vi "PID Calibrator main.vi"() -> ()   [LabVIEW 2021]
panel:
  out "error out":errorcluster
  out "Waveform Chart":T1(graph)
  out "Numeric":i32
  out "remote port":u16
  out "remote address":string
  in  "stop":bool
  in  "port":u16
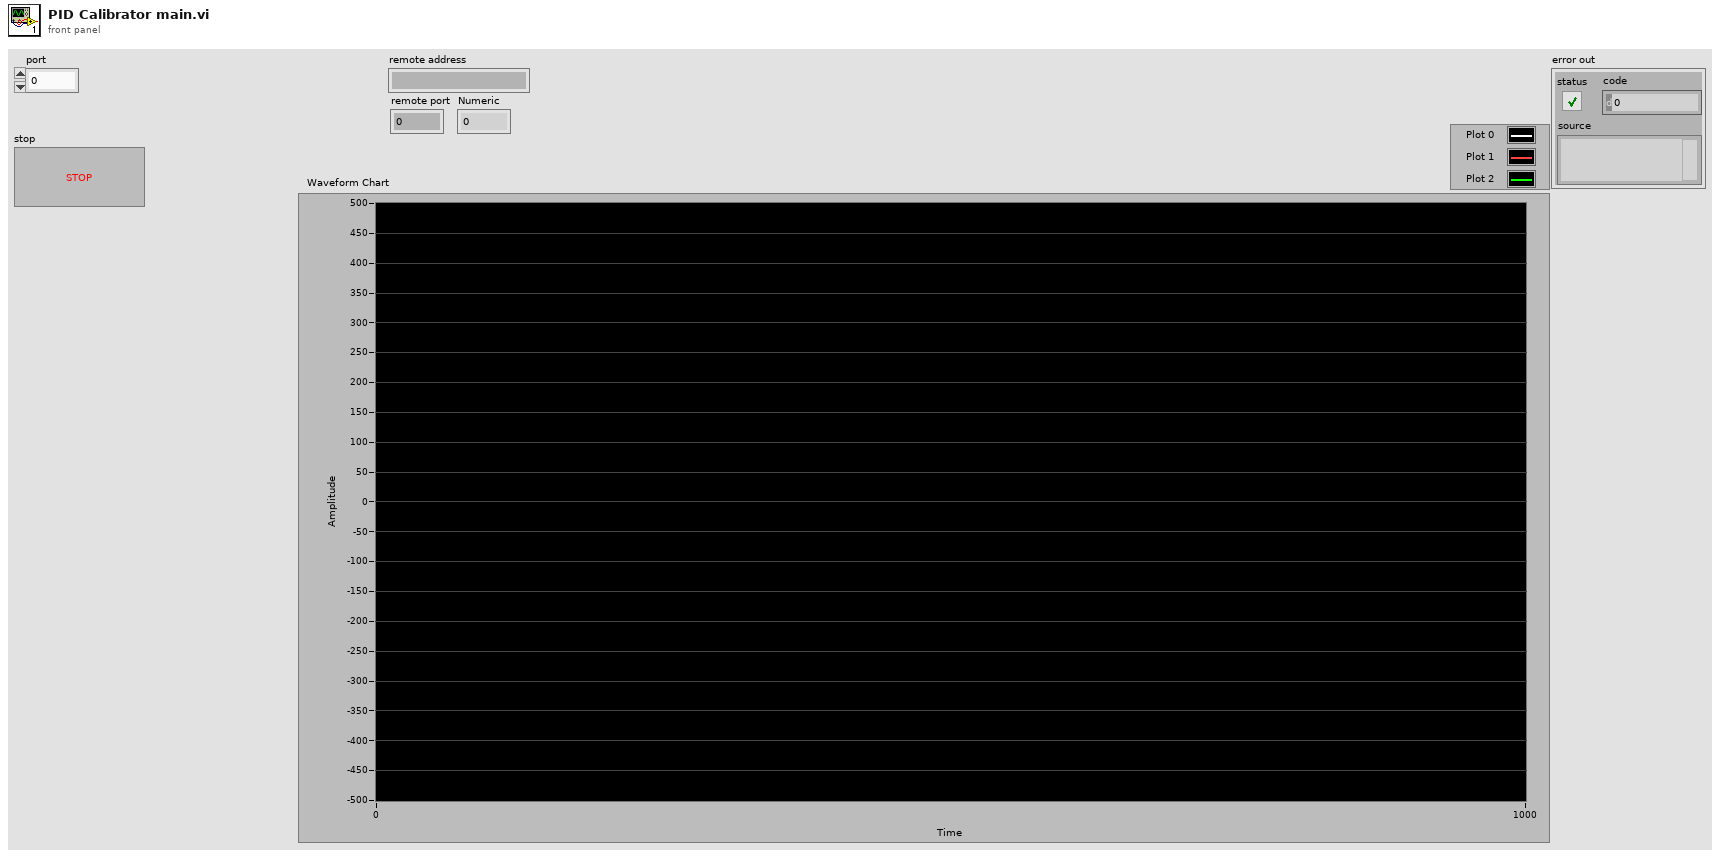
[diagram p1: front panel]
types:
  T1 = cluster{"leftWheelSpeed":dbl, "rightWheelSpeed":dbl, "sonarDistance":dbl}
  T2 = enum16{"Standard", "Buffered", "CRLF", "Immediate"}
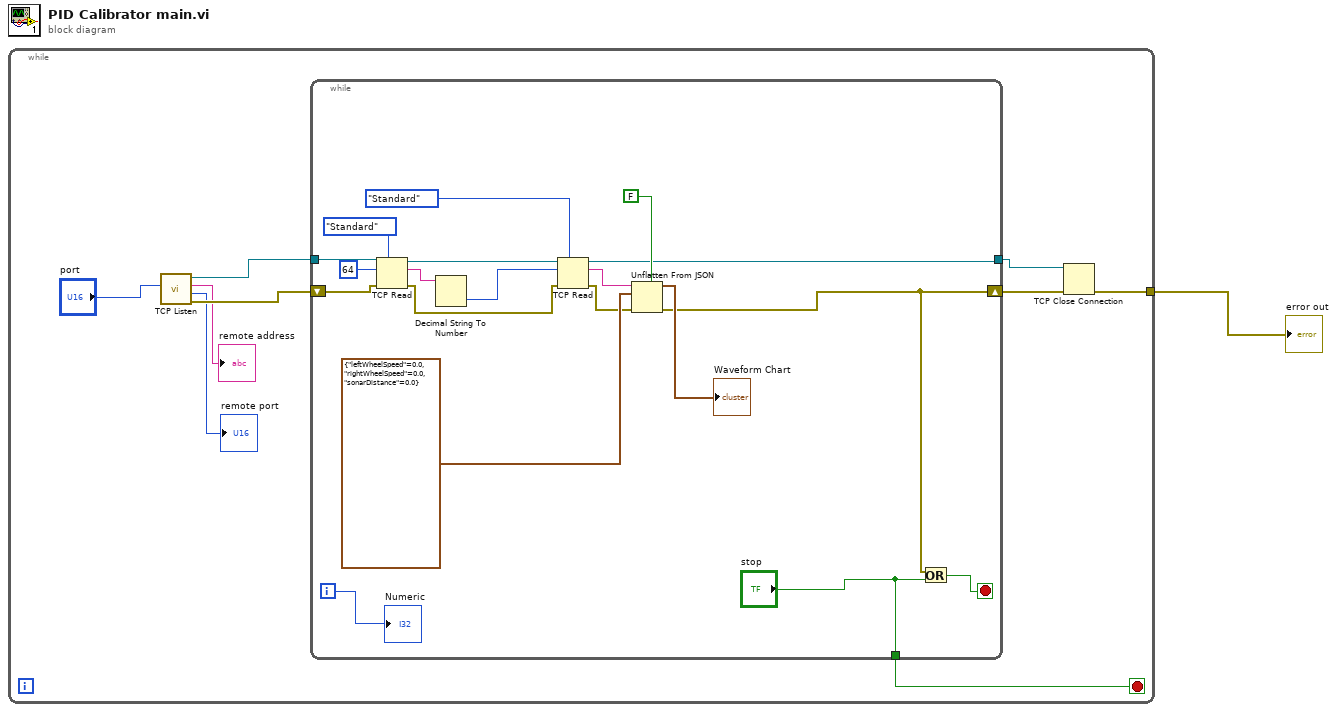
[diagram p0: block diagram]
diagram:
  n1 = while {
    tunnel: [w2] -> w1
    stop <- w3 stop-if-true
    n2 = call <vilib>:"TCP Listen.vi"("port"="port") -> ("error out"=w8:errorcluster, "remote port"=→"remote port":u16, "remote address"=→"remote address":string, "connection ID"=w9:refnum<k5>)  [unwired: 6 in, 1 out]
    n3 = while {
      tunnel: w9 -> [w29]
      tunnel: [w20] -> w7
      shift-right: [w12] -> w6
      shift-left: w8 -> [w14]
      tunnel: ["stop"] -> w3
      i -> [w24]
      stop <- w13 stop-if-true
      n4 = TCP Read(connection ID=w29, bytes to read=64, error in (no error)=w14, 7:T2."Standard" ("mode (standard)")) -> (connection ID out=w23:refnum<k5>, data out=w19:string, error out=w16:errorcluster)  [unwired: 1 in]
      n5 = Decimal String To Number(string=w19) -> (number=w18:i32)  [unwired: 2 in, 1 out]
      n6 = TCP Read(connection ID=w23, bytes to read=w18, error in (no error)=w16, 7:T2."Standard" ("mode (standard)")) -> (connection ID out=w20:refnum<k5>, data out=w21:string, error out=w15:errorcluster)  [unwired: 1 in]
      n7 = Unflatten From JSON(enable LabVIEW extensions? (T)=FALSE, JSON string=w21, type and defaults=T1 {"leftWheelSpeed"=0.0, "rightWheelSpeed"=0.0, "sonarDistance"=0.0}, error in (no error)=w15) -> (value=→"Waveform Chart":T1, error out=w12:errorcluster)  [unwired: 3 in]
      n8 = Or(x=w12, y="stop") -> (x .or. y?=w13:bool)
      "Numeric" <- w24
    }
    n9 = TCP Close Connection(connection ID=w7, error in (no error)=w6) -> (error out=w2:errorcluster)  [unwired: 1 in, 1 out]
  }
  "error out" <- w1
